vi "GOOP_ARGBToRGB.vi"(0 "ARGB":u32 format="%06x", 7 "BackgroundColor":u32(colorbox), 11 "error in":errorcluster) -> (4 "RGB":u32 format="%06x", 15 "error out":errorcluster)   [LabVIEW 2020]
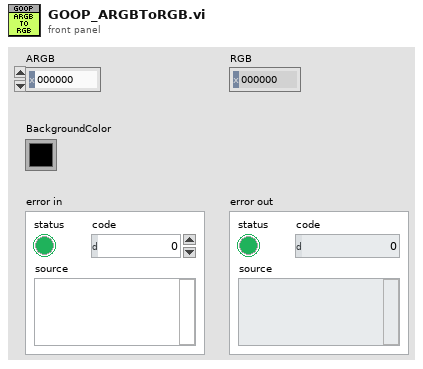
[diagram p1: front panel]
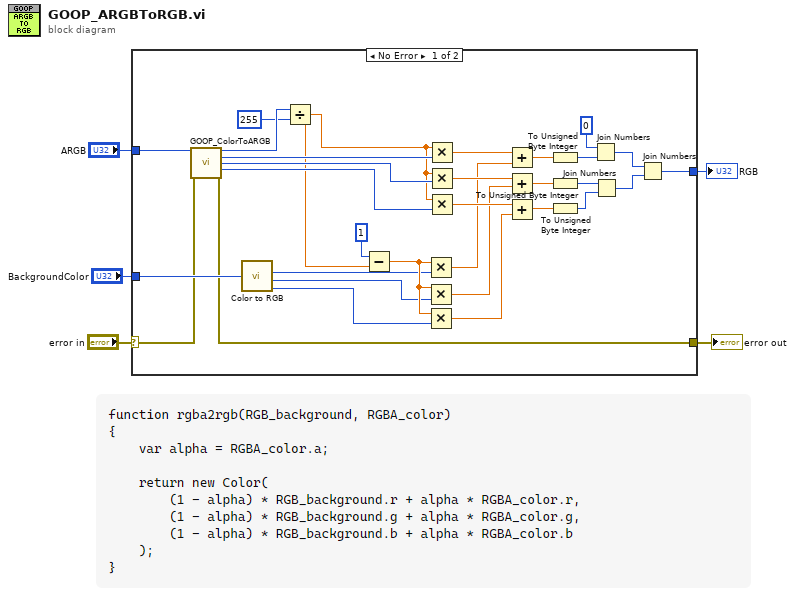
[diagram p0: block diagram]
diagram:
  n1 = case shown="No Error" "error in" {
    selector: "error in" -> [w32 w37]
    tunnel: [w34 w37] -> w4
    tunnel: "BackgroundColor" -> [w36 _]
    tunnel: "ARGB" -> [w33 _]
    tunnel: [w35 _] -> w1
    frame No Error {
      n2 = call "GOOP_ColorToARGB.vi"("Color"=w33, "error in"=w32) -> ("A"=w26:u8, "R"=w29:u8, "G"=w28:u8, "B"=w27:u8, "error out"=w34:errorcluster)  [unwired: 9 in]
      n3 = call <vilib>:"Color to RGB.vi"("Color"=w36) -> ("R"=w25:u8, "G"=w24:u8, "B"=w23:u8)  [unwired: 1 out]
      n4 = Divide(x=w26, y=u8 255) -> (x/y=w7:dbl)
      n5 = Subtract(x=1, y=w7) -> (x-y=w31:dbl)
      n6 = Multiply(x=w31, y=w25) -> (x*y=w19:dbl)
      n7 = Multiply(x=w31, y=w24) -> (x*y=w18:dbl)
      n8 = Multiply(x=w31, y=w23) -> (x*y=w17:dbl)
      n9 = Multiply(x=w7, y=w29) -> (x*y=w22:dbl)
      n10 = Multiply(x=w7, y=w28) -> (x*y=w21:dbl)
      n11 = Multiply(x=w7, y=w27) -> (x*y=w20:dbl)
      n12 = Add(x=w22, y=w19) -> (x+y=w16:dbl)
      n13 = Add(x=w21, y=w18) -> (x+y=w14:dbl)
      n14 = Add(x=w20, y=w17) -> (x+y=w13:dbl)
      n15 = To Unsigned Byte Integer(number=w16) -> (unsigned 8bit integer=w10:u8)
      n16 = To Unsigned Byte Integer(number=w14) -> (unsigned 8bit integer=w9:u8)
      n17 = To Unsigned Byte Integer(number=w13) -> (unsigned 8bit integer=w8:u8)
      n18 = Join Numbers(hi=u8 0, lo=w10) -> ((hi.lo)=w12:u16)
      n19 = Join Numbers(hi=w9, lo=w8) -> ((hi.lo)=w11:u16)
      n20 = Join Numbers(hi=w12, lo=w11) -> ((hi.lo)=w35:u32)
    }
    frame Error {
    }
  }
  "error out" <- w4
  "RGB" <- w1
